vi "DAC Bringup Step.vi"(5 "start label":string, 7 "waveform name":string, 8 "error in":errorcluster, 11 "Digital session":refnum<k15>) -> (0 "error out":errorcluster, 3 "Digital session out":refnum<k15>)   [LabVIEW 2021]
uses:
  <instrlib>/niDigital/niDigital.llb/niDigital Write Source Waveform (Broadcast U32).vi
  <instrlib>/niDigital/niDigital.llb/niDigital Burst Pattern (Pass Fail).vi
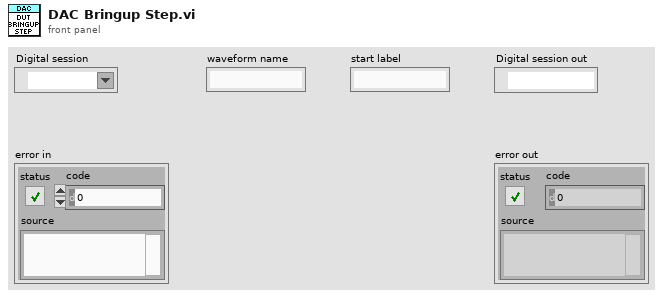
[diagram p1: front panel]
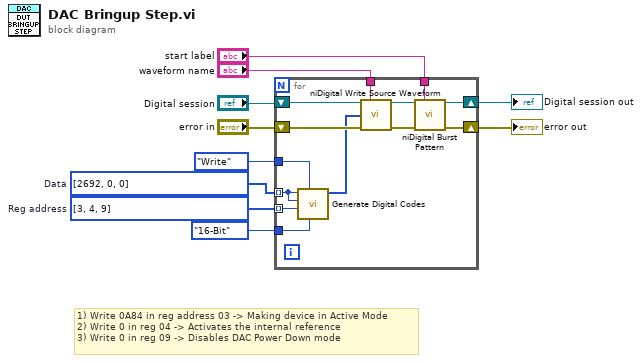
[diagram p0: block diagram]
diagram:
  w3 = u8[] [3, 4, 9]  # Reg address
  w4 = u16[] [2692, 0, 0]  # Data
  # "1) Write 0A84 in reg address 03 -> Making device in Active Mode\n2) Write 0 in reg 04 -> Activates the internal reference\n3) Write 0 in reg 09 -> Disables DAC Power Down mode"
  n1 = for {
    tunnel: "start label" -> [w17]
    tunnel: "waveform name" -> [w16]
    shift-right: [w19] -> w5
    shift-left: "Digital session" -> [w21]
    shift-right: [w18] -> w6
    shift-left: "error in" -> [w20]
    tunnel: w4 -> [w12] mode=indexing
    tunnel: w3 -> [w11] mode=indexing
    tunnel: enum16{"16-Bit", "12-Bit"}."16-Bit" ("Input Code Bit") -> [w14]
    tunnel: enum16{"Read", "Write"}."Write" ("Command") -> [w13]
    n2 = call "Generate Digital Codes.vi"("Input Code Bit"=w14, "Command"=w13, "Address"=w11, "End code"=w12, "Start code"=w12) -> ("Digital commands"=w15:i16[])  [unwired: 4 in, 2 out]
    n3 = call-poly <instrlib>:"niDigital Write Source Waveform.vi"("instrument handle"=w21, "waveform name"=w16, "waveform data"=w15, "error in"=w20) -> ("instrument handle out"=w23:refnum<k15>, "error out"=w22:errorcluster)  [unwired: 10 in]
    n4 = call-poly <instrlib>:"niDigital Burst Pattern.vi"("instrument handle"=w23, "start label"=w17, "error in"=w22) -> ("instrument handle out"=w19:refnum<k15>, "error out"=w18:errorcluster)  [unwired: 10 in, 1 out]
  }
  "error out" <- w6
  "Digital session out" <- w5
